vi "Connect to Simple Web Server.vi"() -> ()   [LabVIEW 2014, in "ESP8266 WiFi Wrapper.lvlib"]
uses:
  ESP8266 WiFi Wrapper.lvlib
  <vilib>/Aledyne-TSXperts/Arduino Compatible Compiler for LabVIEW/Arduino Compatible Compiler for LabVIEW.lvlib
panel:
  in  "Connect to IP":u8[](array[numeric])=[192, 168, 0, 42]
  in  "DNS":u8[](array[numeric])=[0, 0, 0, 0]
  in  "IP address":u8[](array[numeric])=[192, 168, 0, 47]
  in  "Gateway":u8[](array[numeric])=[192, 168, 0, 1]
  in  "Subnet mask":u8[](array[numeric])=[255, 255, 255, 0]
  in  "Password":string="12345678"
  in  "SSID":string="ESP8266 Wifi Example"
  in  "error in (no error)":errorcluster
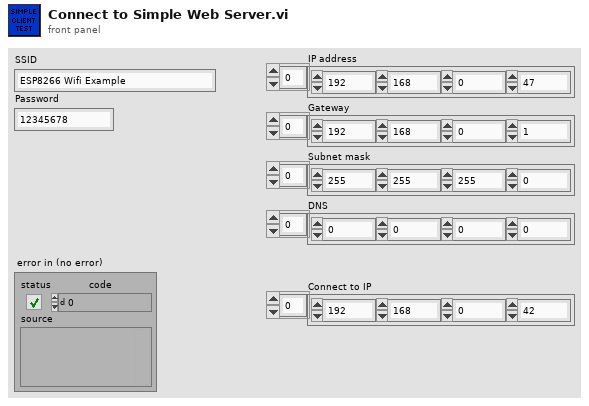
[diagram p1: front panel]
types:
  T1 = enum16{"WIFI_OFF", "WIFI_STA", "WIFI_AP", "WIFI_AP_STA"}
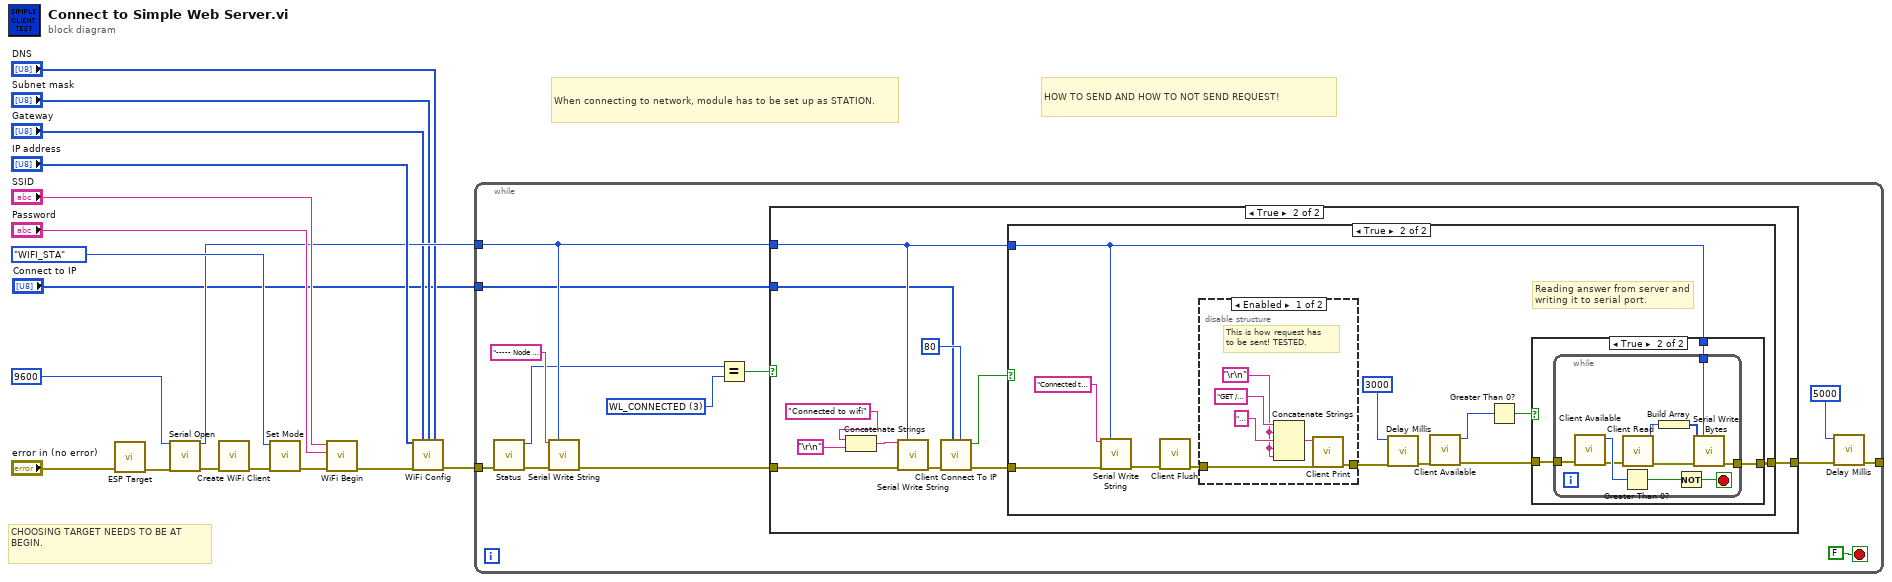
[diagram p0: block diagram]
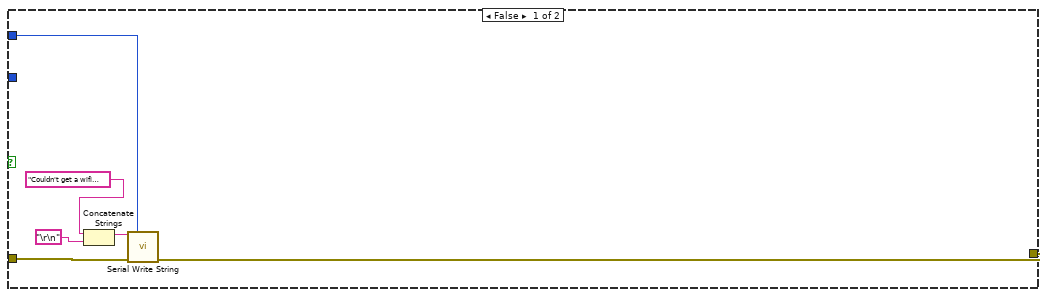
[diagram p2: hidden frame]
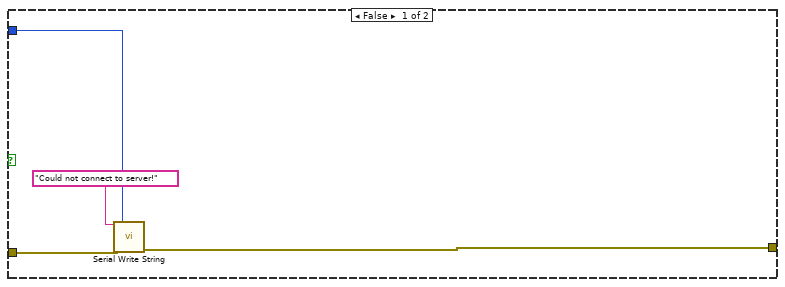
[diagram p3: hidden frame]
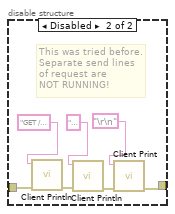
[diagram p4: hidden frame]
diagram:
  # "CHOOSING TARGET NEEDS TO BE AT BEGIN."
  # "When connecting to network, module has to be set up as STATION."
  # "HOW TO SEND AND HOW TO NOT SEND REQUEST!"
  n1 = call "ESP Target.vi"("Error In"="error in (no error)") -> ("Error Out"=w2:errorcluster)  [unwired: 10 in]
  n2 = call <vilib>:"Serial Open.vi"("Speed"=u32 9600, "error in (no error)"=w2) -> ("Instance"=w10:u8, "error out"=w9:errorcluster)  [unwired: 12 in]
  n3 = call "Create WiFi Client.vi"("Error In"=w9) -> ("Error Out"=w8:errorcluster)  [unwired: 10 in]
  n4 = call "Set Mode.vi"("Error In"=w8, "WiFi Server Mode"=T1."WIFI_STA") -> ("Error Out"=w13:errorcluster)  [unwired: 9 in]
  n5 = call "WiFi Begin.vi"("Error In"=w13, "Password"="Password", "SSID"="SSID") -> ("Error Out"=w11:errorcluster)  [unwired: 8 in]
  n6 = call "WiFi Config.vi"("IP address"="IP address", "Gateway address"="Gateway", "Subnet mask"="Subnet mask", "DNS address"="DNS", "Error In"=w11) -> ("Error Out"=w7:errorcluster)  [unwired: 10 in]
  n7 = while {
    tunnel: w10 -> [w25]
    tunnel: w7 -> [w29]
    tunnel: [w19] -> _
    tunnel: "Connect to IP" -> [w18]
    stop <- FALSE stop-if-true
    w23 = u8 3 items=["WL_NO_SHIELD"=255, "WL_IDLE_STATUS"=0, "WL_NO_SSID_AVAIL"=1, "WL_SCAN_COMPLETED"=2, "WL_CONNECTED"=3, "WL_CONNECT_FAILED"=4, "WL_CONNECTION_LOST"=5, "WL_DISCONNECTED"=6] ("Ring")
    n8 = call "Status.vi"("Error In"=w29) -> ("Error Out"=w27:errorcluster, "Status"=w22:u8)  [unwired: 9 in]
    n9 = call <vilib>:"Serial Write String.vi"("String"="----- Node 1 --------", "Instance"=w25, "error in (no error)"=w27) -> ("error out"=w26:errorcluster)  [unwired: 12 in]
    n10 = Equal?(x=w22, y=w23) -> (x = y?=w24:bool)
    n11 = case shown="True" w24 {
      tunnel: [w31 w38] -> w20
      tunnel: w25 -> [w36 w46]
      tunnel: w26 -> [w35 w47]
      tunnel: w18 -> [_ w37]
      frame False {
        n12 = Concatenate Strings("Couldn't get a wifi connection" ("String"), "\r\n" ("End of Line Constant")) -> (w32:string)
        n13 = call <vilib>:"Serial Write String.vi"("String"=w32, "Instance"=w36, "error in (no error)"=w35) -> ("error out"=w31:errorcluster)  [unwired: 12 in]
      }
      frame True {
        n14 = Concatenate Strings("Connected to wifi" ("String"), "\r\n" ("End of Line Constant")) -> (w41:string)
        n15 = call <vilib>:"Serial Write String.vi"("String"=w41, "Instance"=w46, "error in (no error)"=w47) -> ("error out"=w45:errorcluster)  [unwired: 12 in]
        n16 = call "Client Connect To IP.vi"("Port"=u32 80, "IP address"=w37, "Error In"=w45) -> ("Error Out"=w43:errorcluster, "Connected?"=w42:bool)  [unwired: 7 in]
        n17 = case shown="True" w42 {
          tunnel: w46 -> [w48 w60]
          tunnel: [w49 w61] -> w38
          tunnel: w43 -> [w50 w62]
          frame False {
            n18 = call <vilib>:"Serial Write String.vi"("String"="Could not connect to server!", "Instance"=w48, "error in (no error)"=w50) -> ("error out"=w49:errorcluster)  [unwired: 12 in]
          }
          frame True {
            # "Reading answer from server and\nwriting it to serial port."
            n19 = call <vilib>:"Serial Write String.vi"("String"="Connected to server.", "Instance"=w60, "error in (no error)"=w62) -> ("error out"=w53:errorcluster)  [unwired: 12 in]
            n20 = call "Client Flush.vi"("Error In"=w53) -> ("Error Out"=w52:errorcluster)  [unwired: 10 in]
            n21 = disable-structure shown="Enabled" {
              disable-tunnel: [w69 w73] -> w58
              disable-tunnel: w52 -> [w64 w75]
              frame Enabled {
                w65 = "\r\n" ("End of Line Constant")
                # "This is how request has\nto be sent! TESTED."
                n22 = Concatenate Strings("GET /hello HTTP/1.0" ("Input String"), w65, "Connection: close" ("Input String"), w65, w65) -> (w68:string)
                n23 = call "Client Print.vi"("Error In"=w64, "Input String"=w68) -> ("Error Out"=w69:errorcluster)  [unwired: 9 in]
              }
              frame Disabled {
                # "This was tried before.\nSeparate send lines\nof request are \nNOT RUNNING!"
                n24 = call "Client Println.vi"("Error In"=w75, "Input String"="GET /hello HTTP/1.0") -> ("Error Out"=w76:errorcluster)  [unwired: 9 in]
                n25 = call "Client Println.vi"("Error In"=w76, "Input String"="Connection: close") -> ("Error Out"=w74:errorcluster)  [unwired: 9 in]
                n26 = call "Client Print.vi"("Error In"=w74, "Input String"="\r\n") -> ("Error Out"=w73:errorcluster)  [unwired: 9 in]
              }
            }
            n27 = call <vilib>:"Delay Millis.vi"("error in (no error)"=w58, "delay"=u32 3000) -> ("error out"=w57:errorcluster)  [unwired: 9 in]
            n28 = call "Client Available.vi"("Error In"=w57) -> ("Error Out"=w56:errorcluster, "Chars to read"=w54:i16)  [unwired: 9 in]
            n29 = Greater Than 0?(x=w54) -> (x > 0?=w55:bool)
            n30 = case shown="True" w55 {
              tunnel: [w77 w80] -> w61
              tunnel: w60 -> [_ w79]
              tunnel: w56 -> [w77 w78]
              frame False {
              }
              frame True {
                n31 = while {
                  tunnel: [w90] -> w80
                  tunnel: w79 -> [w89]
                  tunnel: w78 -> [w88]
                  stop <- w86 stop-if-true
                  n32 = call "Client Available.vi"("Error In"=w88) -> ("Error Out"=w84:errorcluster, "Chars to read"=w85:i16)  [unwired: 9 in]
                  n33 = Greater Than 0?(x=w85) -> (x > 0?=w87:bool)
                  n34 = call "Client Read.vi"("Error In"=w84) -> ("Error Out"=w83:errorcluster, "Read char"=w82:u8)  [unwired: 9 in]
                  n35 = Build Array(w82) -> (w81:u8[])
                  n36 = Not(x=w87) -> (.not. x?=w86:bool)
                  n37 = call <vilib>:"Serial Write Bytes.vi"("Data"=w81, "Instance"=w89, "error in (no error)"=w83) -> ("error out"=w90:errorcluster)  [unwired: 12 in]
                }
              }
            }
          }
        }
      }
    }
    n38 = call <vilib>:"Delay Millis.vi"("error in (no error)"=w20, "delay"=u32 5000) -> ("error out"=w19:errorcluster)  [unwired: 9 in]
  }
